vi "MGI Decimate Array with Offset (SGL[][][][]).vi"(7 "Array Index(0-3)":i32, 8 "error in (no error)":errorcluster, 9 "Offset":i32, 10 "Decimation":i32, 11 "Single[][][][] In":sgl[][][][](array[numeric])) -> (0 "error out":errorcluster, 3 "Single[][][][] Out":sgl[][][][](array[numeric]))   [LabVIEW 2016]
doc: "Decimates the specified array by the specified amount. An error is output if the array length is not an integer multiple of the decimation. \"Offset\" specifies which decimation is output. An error is output if Offset is greater than or equal to the Decimation.\n\n\nAuthored by Shawn Walpole\nsupport@mooregoodideas.com\nwww.mooregoodideas.com\n\nCopyright (c) 2010, Moore Good Ideas, Inc.\n\nAll rights reserved.\n\nRedistribution and use in source and binary forms, with or without modification, are permitted provided that the following conditions are met:\n\n * Redistributions of source code must retain the above copyright notice, this list of conditions and the following disclaimer.\n * Redistributions in binary form must reproduce the above copyright notice, this list of conditions and the following disclaimer in the documentation and/or other materials provided with the distribution.\n * Neither the name of Moore Good Ideas, Inc. nor the names of its contributors may be used to endorse or promote products derived from this software without specific prior written permission.\n\nTHIS SOFTWARE IS PROVIDED BY THE COPYRIGHT HOLDERS AND CONTRIBUTORS \"AS IS\" AND ANY EXPRESS OR IMPLIED WARRANTIES, INCLUDING, BUT NOT LIMITED TO, THE IMPLIED WARRANTIES OF MERCHANTABILITY AND FITNESS FOR A PARTICULAR PURPOSE ARE DISCLAIMED. IN NO EVENT SHALL THE COPYRIGHT OWNER OR CONTRIBUTORS BE LIABLE FOR ANY DIRECT, INDIRECT, INCIDENTAL, SPECIAL, EXEMPLARY, OR CONSEQUENTIAL DAMAGES (INCLUDING, BUT NOT LIMITED TO, PROCUREMENT OF SUBSTITUTE GOODS OR SERVICES; LOSS OF USE, DATA, OR PROFITS; OR BUSINESS INTERRUPTION) HOWEVER CAUSED AND ON ANY THEORY OF LIABILITY, WHETHER IN CONTRACT, STRICT LIABILITY, OR TORT (INCLUDING NEGLIGENCE OR OTHERWISE) ARISING IN ANY WAY OUT OF THE USE OF THIS SOFTWARE, EVEN IF ADVISED OF THE POSSIBILITY OF SUCH DAMAGE."
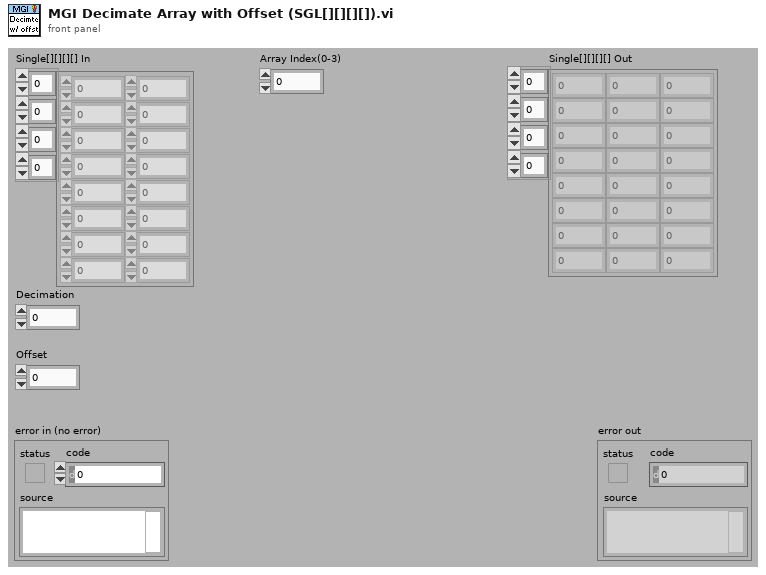
[diagram p1: front panel]
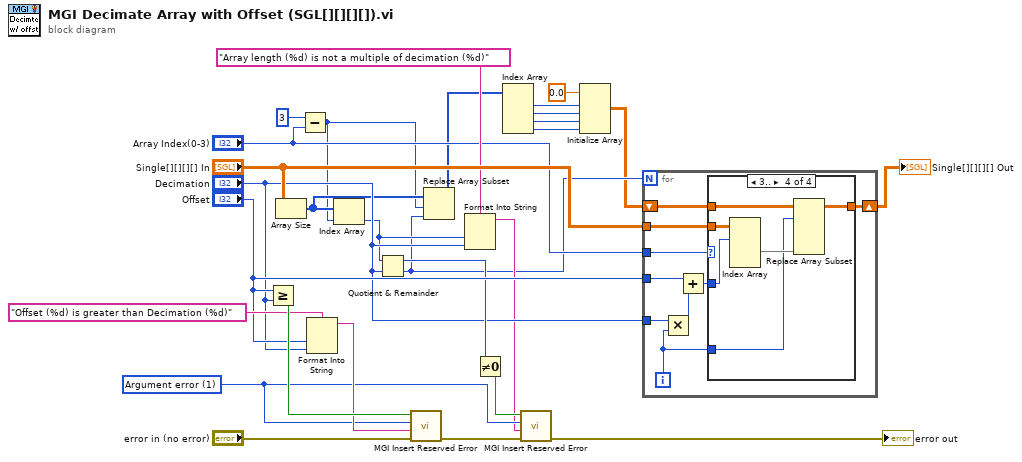
[diagram p0: block diagram]
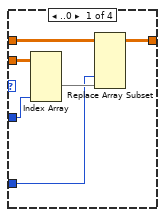
[diagram p2: hidden frame]
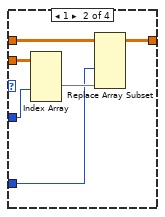
[diagram p3: hidden frame]
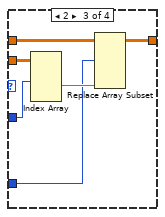
[diagram p4: hidden frame]
diagram:
  w19 = u16 1 items=["No error", "Argument error", "Memory is full", "Out of zone", "End of file", "File already open", "Generic file I/O error", "File not found", "File permission error", "Disk is full", "Duplicate path", "Too many files open", "System feature not enabled", "Resource file not found", "Cannot add resource", "Resource not found", "Image not found", "Image memory error", "Pen does not exist", "Config type invalid", "Config token not found", "Config parse error", "Config memory error", "Bad external code format", "Bad external code offset", "External code not present", "Null window", "Destroy window error", "Null menu", "Print aborted", "Bad print record", "Print driver error", "Windows error during printing", "Memory error during printing", "Print dialog error", "Generic print error", "Invalid device refnum", "Device not found", "Device parameter error", "Device unit error", "Cannot open device", "Device call aborted", "Generic error", "Cancelled by user", "Object ID too low", "Object ID too high", "Object not in heap", "Unknown heap", "Unknown object (invalid DefProc)", "Unknown object (DefProc not in table)", "Message out of range", "Invalid (null) method", "Unknown message", "Manager call not supported", "Bad address", "Network operation in progress", "Network operation timed out", "Connection is busy", "Network attribute not supported", "Network error", "Address in use", "System out of memory", "Connection aborted", "Connection refused", "Not connected", "Already connected", "Connection closed", "Initialization error (interapplication manager)", "Bad occurrence", "Wait on unbound occurrence handler", "Occurrence queue overflow", "Datalog type conflict", "Unused", "Unrecognized type (interapplication manager)", "Memory corrupt", "Failed to make temporary DLL", "Old CIN version", "Drag socket not found", "Failed to load drop-object", "Failed to register OLE object", "Failed to release OLE object", "Format specifier type mismatch", "Unknown format specifier", "Too few format specifiers", "Too many format specifiers", "Scan failed", "Newer CIN version", "OLE Convert", "Runtime menu error", "Password tampered", "Unknown error code"] ("Reserved Error Code")
  n1 = Greater Or Equal?(x="Offset", y="Decimation") -> (x >= y?=w26:bool)
  n2 = Array Size(array="Single[][][][] In") -> (size(s)=w10:i32[])
  n3 = Subtract(x=3 ("y"), y="Array Index(0-3)") -> (x-y=w9:i32)
  n4 = Format Into String(format string="Offset (%d) is greater than Decimation (%d)", "Offset", "Decimation") -> (resulting string=w23:string)  [unwired: 2 in, 1 out]
  n5 = Index Array(array=w10, index=w9) -> (element=w13:i32)
  n6 = Quotient & Remainder(x=w13, y="Decimation") -> (x-y*floor(x/y)=w18:i32, floor(x/y)=w8:i32)
  n7 = call <userlib>:"MGI Insert Reserved Error.vi"("Error In"="error in (no error)", "Error Description"=w23, "Reserved Error Code (Generic error)"=w19, "Error? (T)"=w26) -> ("Error Out"=w21:errorcluster)  [unwired: 7 in]
  n8 = Replace Array Subset(array=w10, new element=w8, index=w9) -> (w7:i32[])
  n9 = Format Into String(format string="Array length (%d) is not a multiple of decimation (%d)", w13, "Decimation") -> (resulting string=w15:string)  [unwired: 2 in, 1 out]
  n10 = Not Equal To 0?(x=w18) -> (x != 0?=w22:bool)
  n11 = Index Array(array=w7) -> (element #1=w6:i32, element #2=w5:i32, element #3=w2:i32, element #4=w1:i32)  [unwired: 4 in]
  n12 = call <userlib>:"MGI Insert Reserved Error.vi"("Error In"=w21, "Error Description"=w15, "Reserved Error Code (Generic error)"=w19, "Error? (T)"=w22) -> ("Error Out"=→"error out":errorcluster)  [unwired: 7 in]
  n13 = Initialize Array(sgl 0.0, w6, w5, w2, w1) -> (w4:sgl[][][][])
  n14 = for {
    N: w8 -> [_]
    tunnel: "Decimation" -> [w37]
    tunnel: "Offset" -> [w36]
    tunnel: "Single[][][][] In" -> [w34]
    tunnel: "Array Index(0-3)" -> [w33]
    shift-right: [w29] -> w3
    shift-left: w4 -> [w31]
    i -> [w30]
    n15 = Multiply(x=w37, y=w30) -> (x*y=w35:i32)
    n16 = Add(x=w36, y=w35) -> (x+y=w32:i32)
    n17 = case shown="3.." w33 {
      tunnel: w34 -> [w43 w49 w55 w61]
      tunnel: w32 -> [w39 w45 w51 w57]
      tunnel: w31 -> [w42 w48 w54 w60]
      tunnel: w30 -> [w38 w44 w50 w56]
      tunnel: [w40 w46 w52 w58] -> w29
      frame ..0 {
        n18 = Index Array(array=w43, index (dim 3)=w39) -> (element=w41:sgl[][][])  [unwired: 3 in]
        n19 = Replace Array Subset(array=w42, new element=w41, index (dim 3)=w38) -> (w40:sgl[][][][])  [unwired: 3 in]
      }
      frame 1 {
        n20 = Index Array(array=w49, index (dim 2)=w45) -> (element=w47:sgl[][][])  [unwired: 3 in]
        n21 = Replace Array Subset(array=w48, new element=w47, index (dim 2)=w44) -> (w46:sgl[][][][])  [unwired: 3 in]
      }
      frame 2 {
        n22 = Index Array(array=w55, index (dim 1)=w51) -> (element=w53:sgl[][][])  [unwired: 3 in]
        n23 = Replace Array Subset(array=w54, new element=w53, index (dim 1)=w50) -> (w52:sgl[][][][])  [unwired: 3 in]
      }
      frame 3.. {
        n24 = Index Array(array=w61, index (dim 0)=w57) -> (element=w59:sgl[][][])  [unwired: 3 in]
        n25 = Replace Array Subset(array=w60, new element=w59, index (dim 0)=w56) -> (w58:sgl[][][][])  [unwired: 3 in]
      }
    }
  }
  "Single[][][][] Out" <- w3
